vi "mtlb simx Read Proximity Sensor.vi"(0 "clientIDandSensorHandle":i32, 1 "detectedSurfaceNormalVector":sgl, 5 "detectionState":string, 7 "detectedPoint":sgl, 9 "detectedObjectHandle":i32, 11 "error in (no error)":errorcluster, 12 "operationMode":i32) -> (3 "detectedSurfaceNormalVector out":sgl, 4 "clientIDandSensorHandle out":i32, 6 "detectionState out":string, 8 "detectedPoint out":sgl, 10 "detectedObjectHandle out":i32, 14 "function return":i32, 15 "error out":errorcluster)   [LabVIEW 2019, in "PXL_V-REP.lvlib"]
doc: "EXTAPI_DLLEXPORT simxInt mtlb_simxReadProximitySensor(simxInt* clientIDandSensorHandle,simxUChar* detectionState,simxFloat* detectedPoint,simxInt* detectedObjectHandle,simxFloat* detectedSurfaceNormalVector,simxInt operationMode);"
uses:
  PXL_V-REP.lvlib
  <userlib>/V-REP/remoteApi.dll
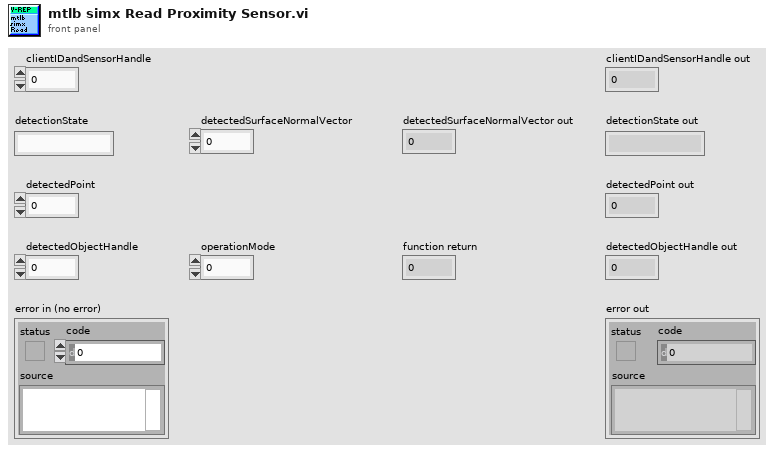
[diagram p1: front panel]
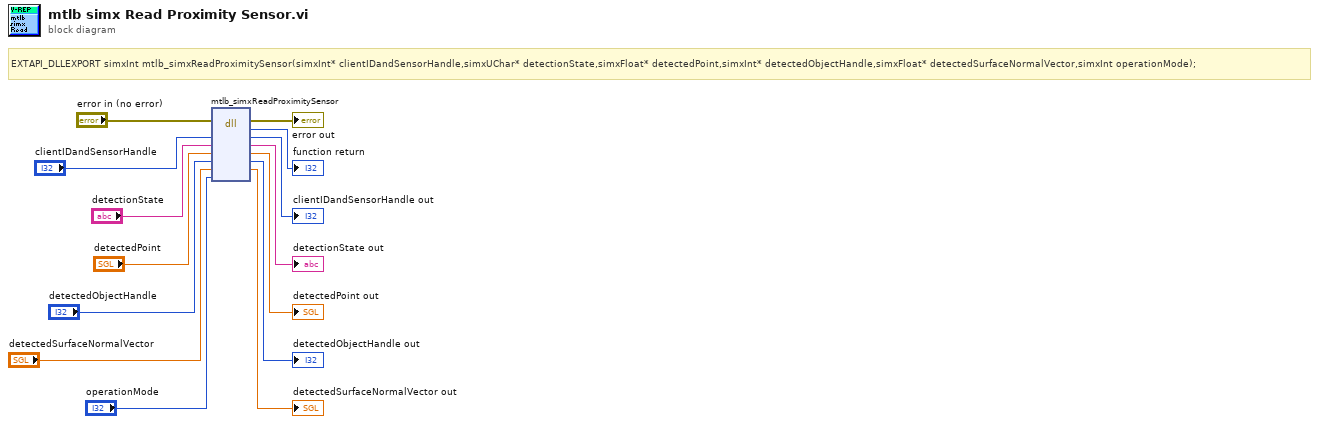
[diagram p0: block diagram]
diagram:
  # "EXTAPI_DLLEXPORT simxInt mtlb_simxReadProximitySensor(simxInt* clientIDandSensorHandle,simxUChar* detectionState,simxFloat* detectedPoint,simxInt* detectedObjectHandle,simxFloat* detectedSurfaceNormalVector,simxInt operationMode);"
  n1 = dll-call lib="C:/Program Files (x86)/National Instruments/LabVIEW 2019/user.lib/V-REP/remoteApi.*" fn="mtlb_simxReadProximitySensor"(error in="error in (no error)", "clientIDandSensorHandle"="clientIDandSensorHandle", "detectionState"="detectionState", "detectedPoint"="detectedPoint", "detectedObjectHandle"="detectedObjectHandle", "detectedSurfaceNormalVector"="detectedSurfaceNormalVector", "operationMode"="operationMode") -> (error out=→"error out":errorcluster, →"function return":i32, "clientIDandSensorHandle"=→"clientIDandSensorHandle out":i32, "detectionState"=→"detectionState out":string, "detectedPoint"=→"detectedPoint out":sgl, "detectedObjectHandle"=→"detectedObjectHandle out":i32, "detectedSurfaceNormalVector"=→"detectedSurfaceNormalVector out":sgl)  [unwired: 3 in, 1 out]
